vi "2002_FireAt1015EveryDay.vi"(8 "error in (no error)":errorcluster) -> (0 "error out":errorcluster)   [LabVIEW 2013]
uses:
  source/Cron.Jenkins/Cron.Jenkins.lvclass/Cron.Jenkins.ctl
  source/Cron.Jenkins/Write Job Name.vi
  <vilib>/addons/_JKI Toolkits/Caraya/classes/Assert/Assert True.vi
  source/Cron/Create Cron Expression.vi
  source/Cron/Compute Next Cron.vi
  source/Cron.Jenkins/Cron.Jenkins.lvclass
  <vilib>/addons/_JKI Toolkits/Caraya/classes/Test/Test.lvclass
  <vilib>/addons/_JKI Toolkits/Caraya/classes/Assert/Assert.lvclass
  source/openCron.lvlib
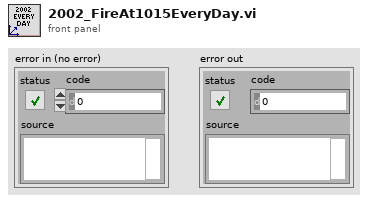
[diagram p1: front panel]
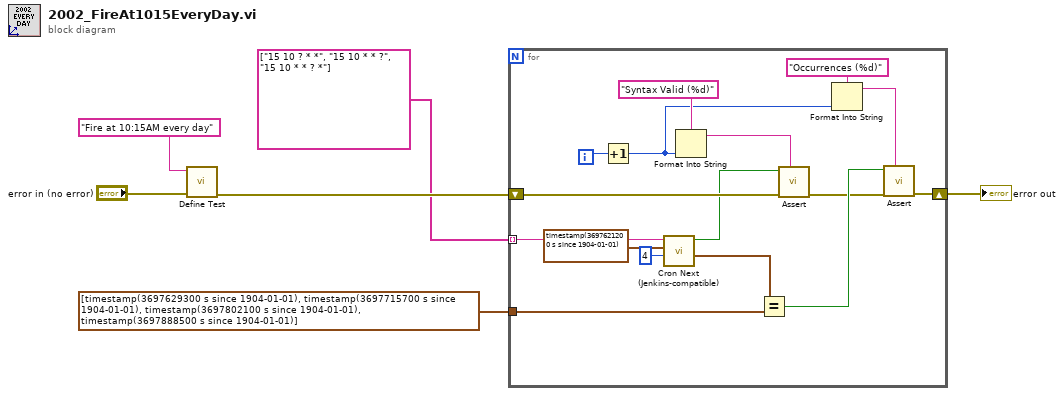
[diagram p0: block diagram]
diagram:
  n1 = call <vilib>:"Define Test.vi"("error in (no error)"="error in (no error)", "Label (VI Title)"="Fire at 10:15AM every day") -> ("error out"=w3:errorcluster)  [unwired: 9 in]
  n2 = for {
    tunnel: timestamp[] [timestamp(3697629300 s since 1904-01-01), timestamp(3697715700 s since 1904-01-01), timestamp(3697802100 s since 1904-01-01), timestamp(3697888500 s since 1904-01-01)] -> [w19]
    tunnel: string[] ["15 10 ? * *", "15 10 * * ?", "15 10 * * ? *"] -> [w11] mode=indexing
    shift-right: [w22] -> w6
    shift-left: w3 -> [w18]
    i -> [w17]
    n3 = Increment(x=w17) -> (x+1=w13:i32)
    n4 = call "Cron Next (Jenkins-compatible).vi"("Nb Occurences (min: 1)"=u16 4, "Reference timestamp (Now)"=timestamp(3697621200 s since 1904-01-01) ("y"), "Cron Expression"=w11) -> ("Occurences"=w8:timestamp[], "syntax valid?"=w7:bool)  [unwired: 6 in, 1 out]
    n5 = Format Into String(format string="Syntax Valid (%d)" ("Label (VI Title)"), w13) -> (resulting string=w15:string)  [unwired: 2 in, 1 out]
    n6 = Equal?(x=w8, y=w19) -> (x = y?=w21:bool)
    n7 = call-poly <vilib>:"Assert.vi"("Label"=w15, "error in (no error)"=w18, "True?"=w7) -> ("error out"=w20:errorcluster)  [unwired: 8 in]
    n8 = Format Into String(format string="Occurrences (%d)" ("Label (VI Title)"), w13) -> (resulting string=w12:string)  [unwired: 2 in, 1 out]
    n9 = call-poly <vilib>:"Assert.vi"("Label"=w12, "error in (no error)"=w20, "True?"=w21) -> ("error out"=w22:errorcluster)  [unwired: 8 in]
  }
  "error out" <- w6
